vi "To-string-array.vi"(8 "error in (no error)":errorcluster, 11 "Action in":refnum<class "Wait.lvclass">) -> (0 "error out":errorcluster, 2 "Action string array":string[](array[string]), 3 "Action out":refnum<class "Wait.lvclass">)   [LabVIEW 2013, in "PowderDeposition.lvlib" / "Wait.lvclass"]
uses:
  Wait.lvclass
  Wait.lvclass/Wait.ctl
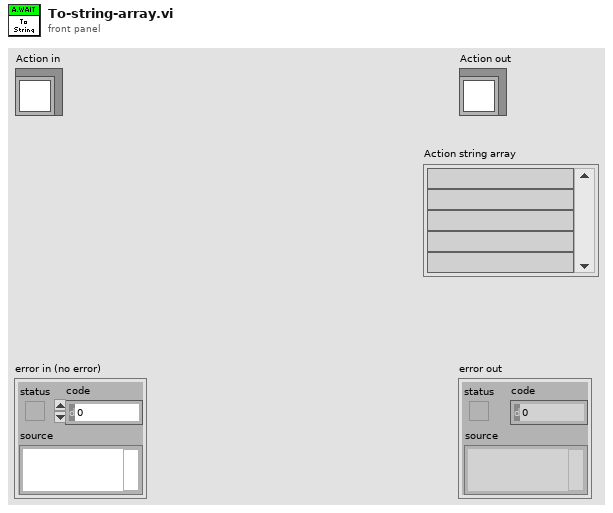
[diagram p1: front panel]
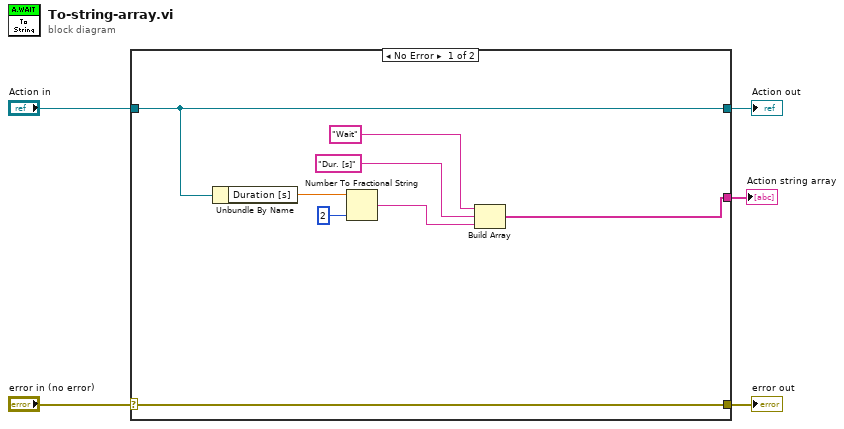
[diagram p0: block diagram]
diagram:
  n1 = case shown="No Error" "error in (no error)" {
    selector: "error in (no error)" -> [w13 w15]
    tunnel: [w13 w15] -> w4
    tunnel: [w12 w14] -> w2
    tunnel: "Action in" -> [w12 w14]
    tunnel: [w7 _] -> w1
    frame No Error {
      n2 = Unbundle By Name(w12) -> ("Duration [s]"=w11:dbl)
      n3 = Number To Fractional String(number=w11, precision (6)=i16 2) -> (F-format string=w9:string)  [unwired: 2 in]
      n4 = Build Array("Wait", "Dur. [s]" ("element"), w9) -> (w7:string[])
    }
    frame Error {
    }
  }
  "error out" <- w4
  "Action out" <- w2
  "Action string array" <- w1
